vi "FPGAmain_5761.vi"() -> ()   [LabVIEW 2018]
uses:
  FPGA/DataMode.ctl
  Host/Scope/controls/host_transfer_speed.ctl
  FPGA/Input_5782/5782_Fast_PID_states.ctl
  <vilib>/Platform/TimedLoop/XDataNode/timing_clust.ctl
  <vilib>/Platform/TimedLoop/XDataNode/nitl_modes.ctl
  <vilib>/Platform/TimedLoop/XDataNode/wakeup.ctl
  <vilib>/rvi/Emulation/niFpgaGetClockAttributes.vi
  <vilib>/rvi/Emulation/niFpgaSctlEmulationGetInTimedLoop.vi
  <vilib>/rvi/Emulation/niFpgaEmulationReportErrorSimple.vi
  <vilib>/rvi/eio/common/nirviEmuTemplateMethod_errors.vi
  <vilib>/rvi/Emulation/niFpgaCriticalErrorInLSC.vi
  <vilib>/rvi/Emulation/niFpgaProcessEmulError.vi
  <vilib>/rvi/Emulation/niFpgaEmulationIsFPGAContextNoSignature.vi
  <vilib>/rvi/errors/niFpgaSetErrorForExecOnDevCompSimple.vi
  <vilib>/rvi/eio/common/nirviEmuReportErrorAndStop.vi
  <vilib>/rvi/DataTransferAndStorage/Container/Common/niFpgaContainerGetUniqueNameForEmu.vi
  <vilib>/rvi/FIFO/Fifo_Resource/nirvififoEmulationSetSize.vi
  <vilib>/rvi/FIFO/Fifo_Resource/nirviFifoEmulationQueueMgr.vi
  <instcachedir>/0/nirviFifoEmulationQueueMgr_E5CAEC123FF24DC58D834DCA3CDAA9B5.lvgen/nirviFifoEmulationQueueMgr_E5CAEC123FF24DC58D834DCA3CDAA9B5_015.vi
  <vilib>/rvi/FIFO/Fifo_Resource/nirvififoEmulationDetermineInputValidOut.vi
  <vilib>/rvi/FIFO/Fifo_Resource/nirvififoEmulationCreateLock.vi
  <vilib>/rvi/FIFO/Fifo_Resource/nirvififoEmulationObtainLock.vi
  <vilib>/rvi/FIFO/Fifo_Resource/nirvififoEmulationReleaseLock.vi
  <vilib>/rvi/occurrence/nirviWaitOnOccurrenceBase.vi
  <vilib>/rvi/errors/nirviReportUnexpectedCaseInternalError.vi
  <vilib>/rvi/errors/nirviReportUnexpectedCaseInternalError (U32).vi
  <vilib>/rvi/Memory/Memory_Emulation/niFpgaMemoryEmulationCacheClearOnFirstRun.vi
  <vilib>/rvi/Memory/Memory_Emulation/nirvimemoryEmulationManagerCache_MakeExclusive.vi
  <vilib>/rvi/Memory/Memory_Emulation/niFpgaMemoryEmulationValidateCache.vi
  <vilib>/rvi/Memory/Memory_Emulation/nirvimemoryEmulationManagerCache_InsertValue.vi
  <vilib>/Utility/error.llb/Clear Errors.vi
  <vilib>/rvi/Memory/Memory_Emulation/nirvimemoryEmulationManagerCache_ReleaseExclusive.vi
  <vilib>/rvi/Memory/Memory_Emulation/nirvimemoryEmulationManagerCache_GetValue.vi
  <vilib>/rvi/Memory/Memory_Emulation/nirvimemoryEmulationManagerCache_SetValue.vi
  <instcachedir>/0/nirviFifoEmulationQueueMgr_E5CAEC123FF24DC58D834DCA3CDAA9B5.lvgen/nirviFifoEmulationQueueMgr_E5CAEC123FF24DC58D834DCA3CDAA9B5_019.vi
  <vilib>/rvi/interface/RandomDataEmulation/niFpgaRandomDataHandleErrors.vi
  <instcachedir>/0/nirviFifoEmulationQueueMgr_E5CAEC123FF24DC58D834DCA3CDAA9B5.lvgen/nirviFifoEmulationQueueMgr_E5CAEC123FF24DC58D834DCA3CDAA9B5_025.vi
  <vilib>/rvi/interface/RandomDataEmulation/nirviRandomDataMultiElementFPGAFIFO.vi
  <instcachedir>/0/nirviRandomDataMultiElementFPGAFIFO_6740B454F3C245F78F76ED91F73FD8DB.lvgen/nirviRandomDataMultiElementFPGAFIFO_6740B454F3C245F78F76ED91F73FD8DB_000.vi
  <vilib>/eio/EIONode/EIONode.xnode
  <vilib>/Platform/TimedLoop/XDataNode/XDataNode.xnode
  <vilib>/rvi/FXPMathLib/FxpInterpret/XNode/nifxpmath_Interpret.xnode
  <vilib>/rvi/DataTransferAndStorage/Container/XNode/niFpgaContainer.xnode
  <vilib>/rvi/FIFO/Fifo_Resource/nirvififoEmulationWrite.vi
  <vilib>/rvi/DataTransferAndStorage/Register/Emulation/niFpgaRegisterEmulation.vi
  <vilib>/rvi/FIFO/Fifo_Resource/nirvififoEmulationRead.vi
  <vilib>/rvi/interface/RandomDataEmulation/nirviRandomDataFpgaReadWriteTemplate.vi
  <vilib>/rvi/interface/RandomDataEmulation/nirviRandomDataFpgaMultiElementTemplate.vi
  <vilib>/Platform/TimedLoop/XDataNode/XDNodeRunTimeDep.lvlib
panel:
  in  "Transfer speed":T1
  out "Num timeout":u32
  in  "W12 enabled":bool
  in  "Sample Clock Commit":bool
  in  "Sample Clock Select":u8
  out "SPI Idle":bool
  out "Configuration Error":bool
  out "Synthesizer Locked":bool
  out "Configured?":bool
  in  "Continuous":bool
  in  "Record length":u16=4000 caption="Samples Per Trigger" min=1 step=1
  in  "Trigger Acquisition":bool
  out "IO Module\\Trigger Input":bool
  in  "Acquisition running":bool
  in  "Simulated phase":fxp<+,64,64>[](array[numeric])=[0.0, 0.0]
  in  "Mode":T2
  in  "Phase input":fxp<+,64,64>[](array[numeric])=[0.0, 0.0, 0.0, 0.0, 0.0, 0.0, 0.0, 0.0, 0.0, 0.0, 0.0, 0.0, 0.0, 0.0, 0.0, 0.0]
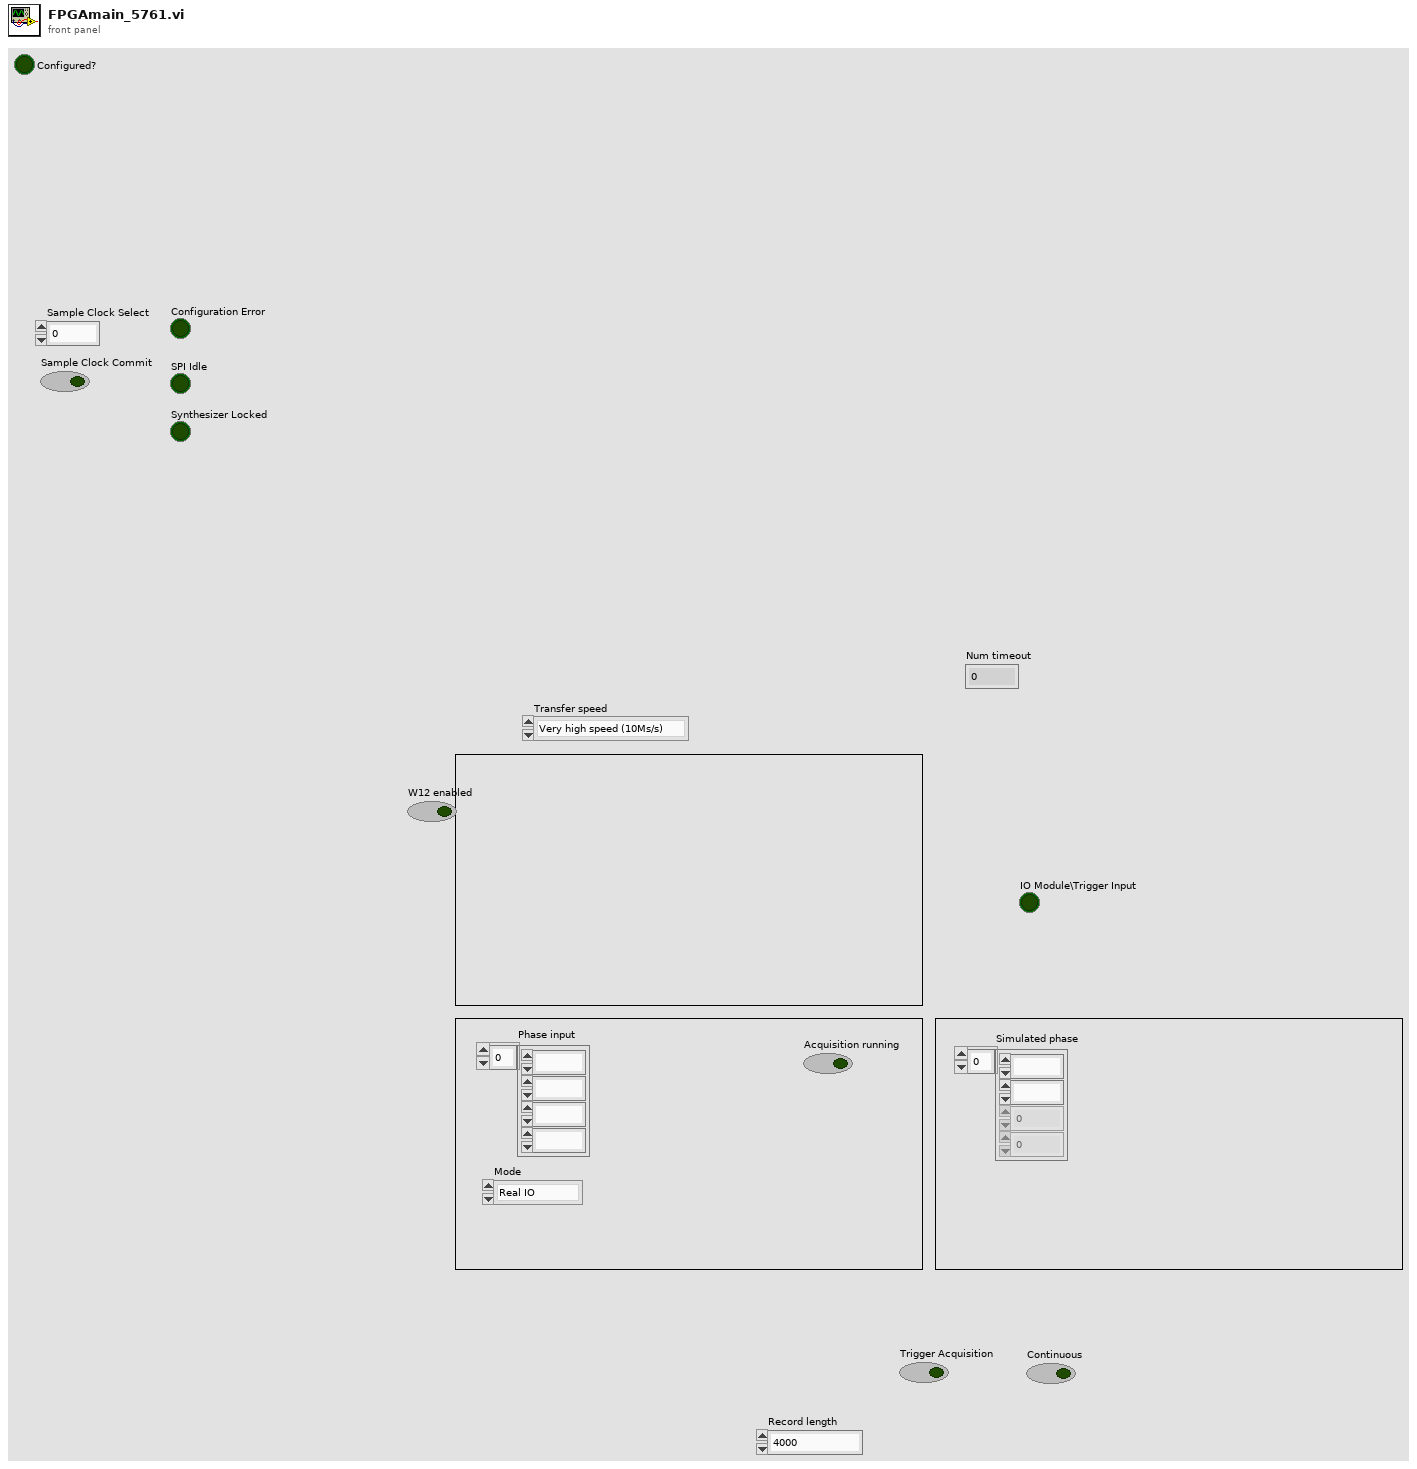
[diagram p1: front panel]
types:
  T1 = typedef "host_transfer_speed.ctl" = enum16{"Very high speed (10Ms/s)", "High speed (1Ms/s)", "Low speed (50kS/s)", "Ultra low speed (20kS/s)"}
  T2 = typedef "DataMode.ctl" = enum16{"Real IO", "Simulated"}
  T3 = typedef "5782_Fast_PID_states.ctl" = enum8{"Wait for trigger", "Acquisition", "Send record length", "Wait for output", "Quiet period"}
  T4 = typedef "XDNodeRunTimeDep.lvlib/timing_clust.ctl" = cluster{"Expected End [f-1]":u64, "Actual End [f-1]":u64, "Finished Late? [f-1]":bool, "Expected End [i-1]":u64, "Actual End [i-1]":u64, "Finished Late? [i-1]":bool, "Expected Start [i]":u64, "Actual Start [i]":u64, "Expected Start [f]":u64, "Actual Start [f]":u64, "Source Name":string, "Structure Name":string, "Period":i64, "Deadline":i64, "Offset":i64, "Start":i64, "Priority":i32, "Timeout":i32, "Mode":T5, "Wakeup Reason":T6, "Error":errorcluster, "Source Type":string, "Secondary Source Type":string, "Global End Time":u64, "Global Start Time":u64, "Frame Duration":u64, "Iteration Duration":u64, "Assigned CPU":i32, "I/O Scan Engine Mode":u32}
  T5 = typedef "XDNodeRunTimeDep.lvlib/nitl_modes.ctl" = enum32{"No Change", "Process missed periods, maintain original phase", "Discard missed periods, maintain original phase", "Process missed periods, ignore original phase", "Discard missed periods, ignore original phase"}
  T6 = typedef "XDNodeRunTimeDep.lvlib/wakeup.ctl" = enum32{"Normal", "Aborted", "Asynchronous wakeup", "Timing source error", "Timed loop error", "Timeout"}
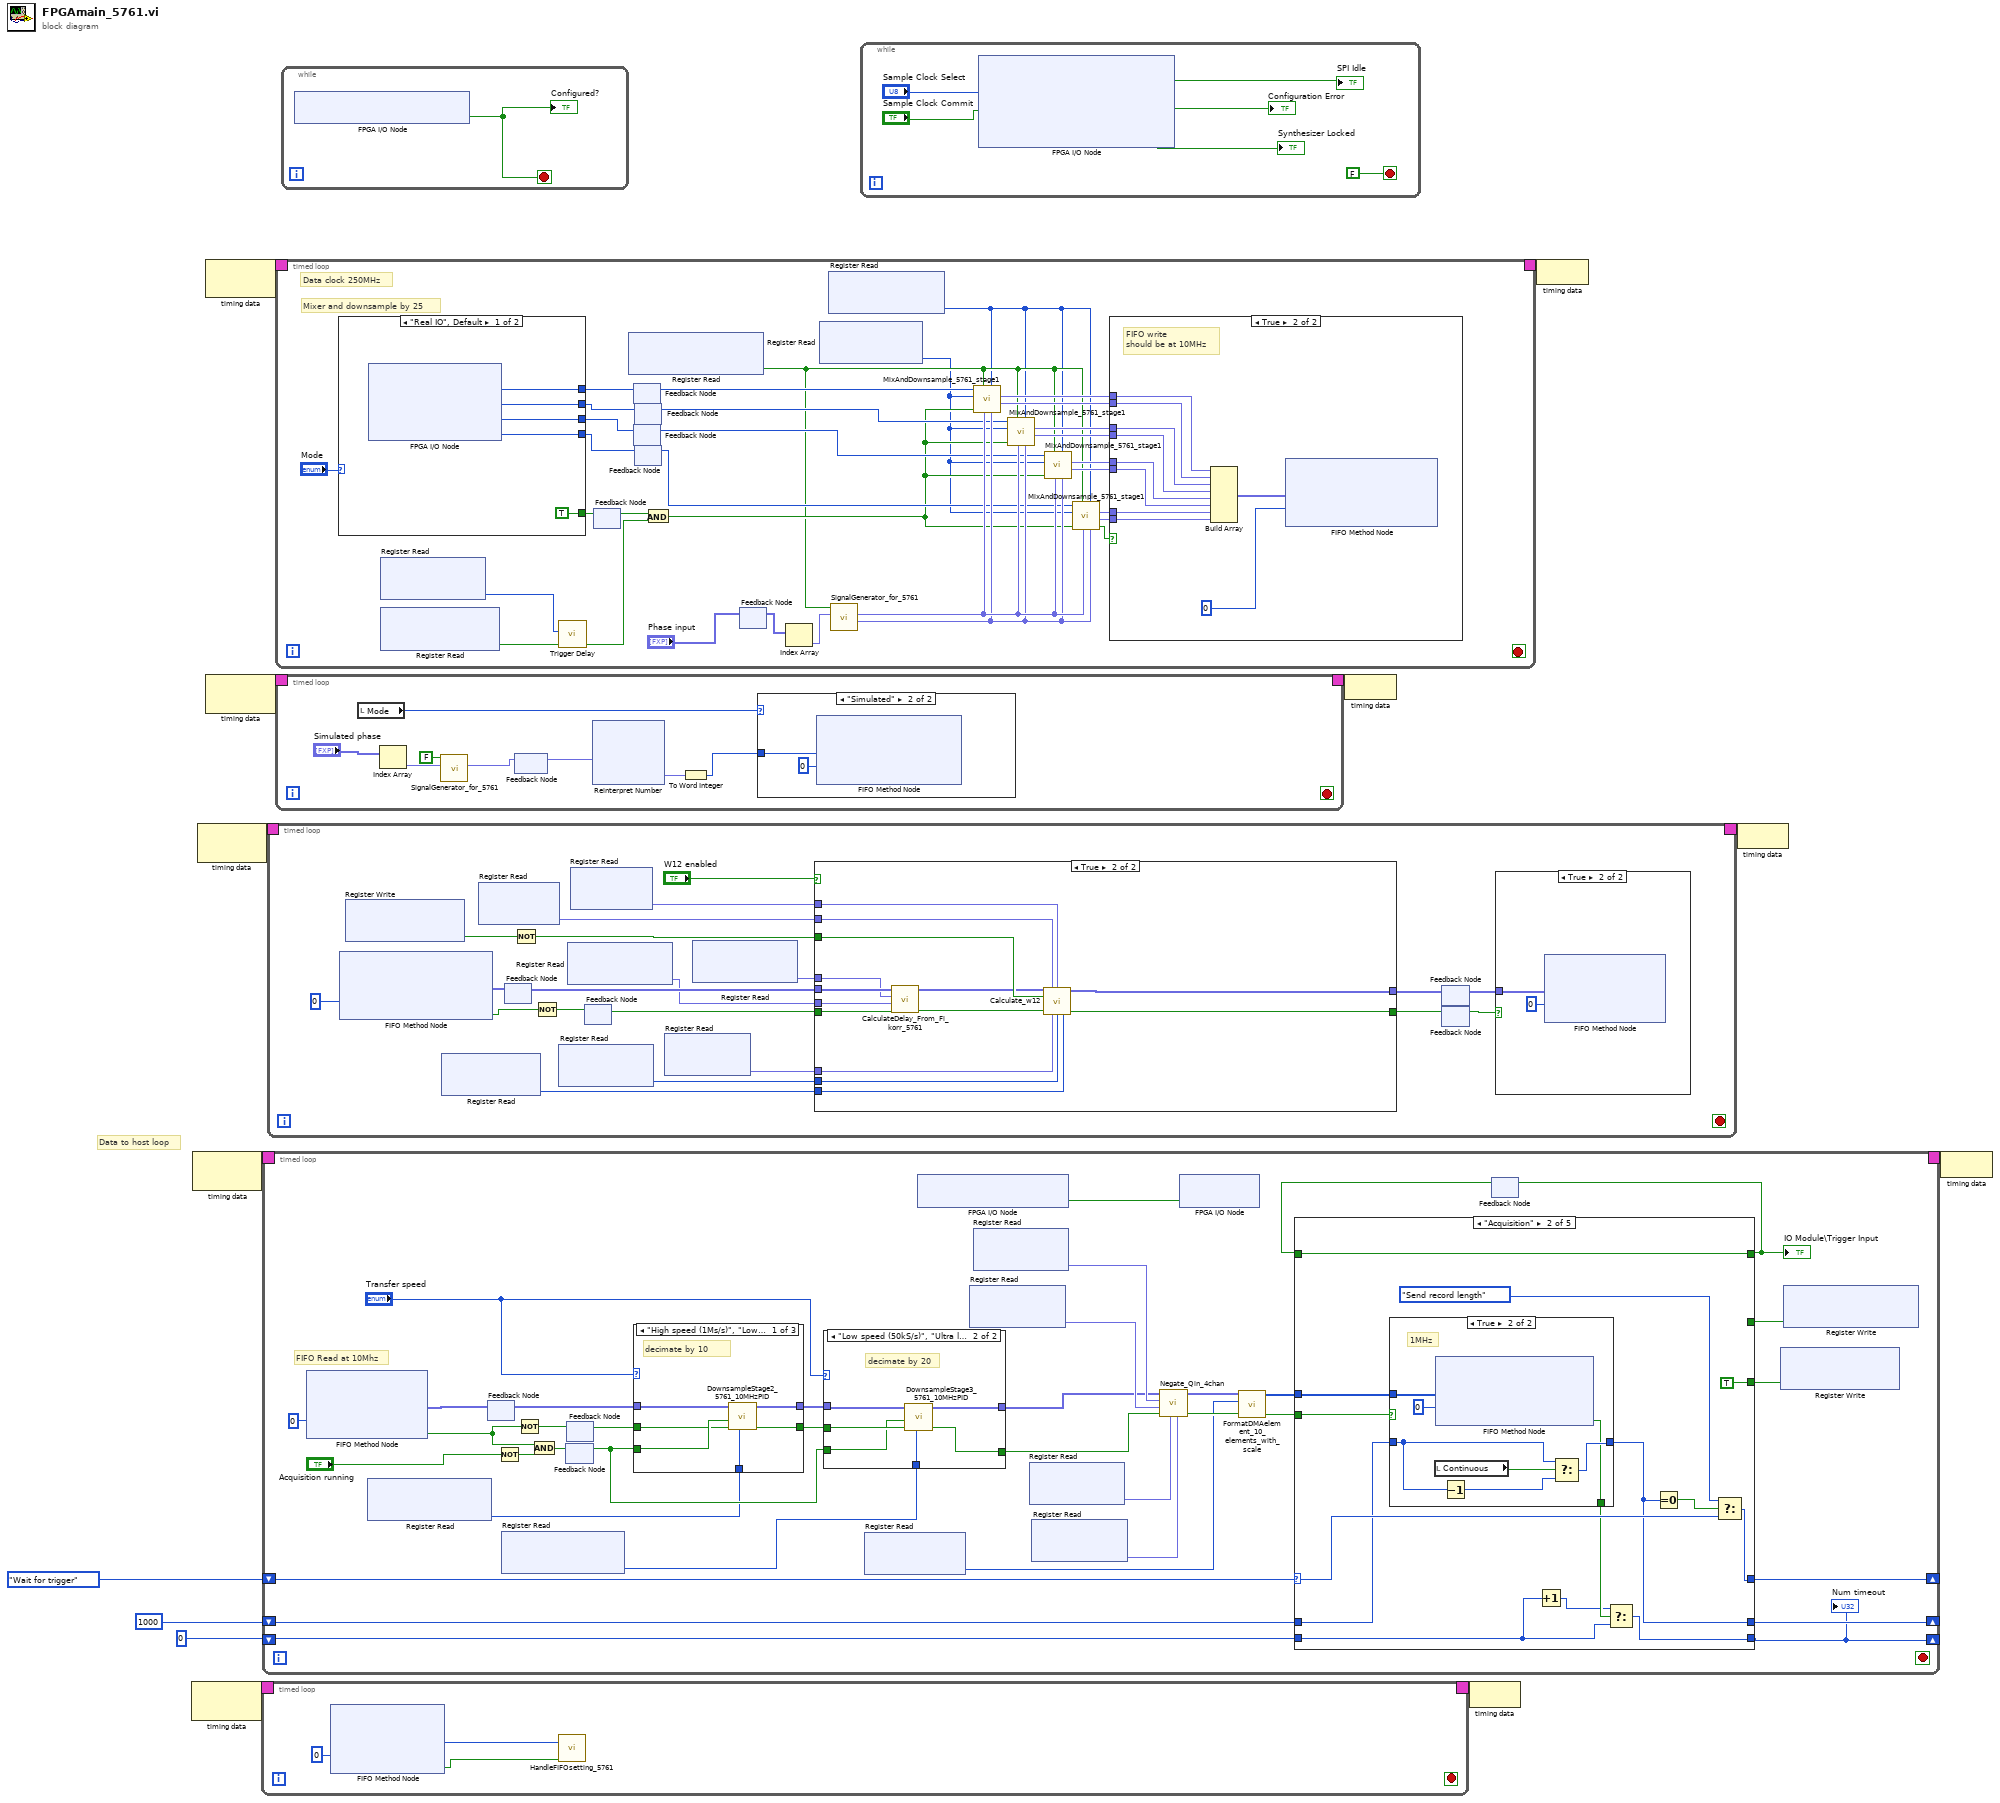
[diagram p0: block diagram]
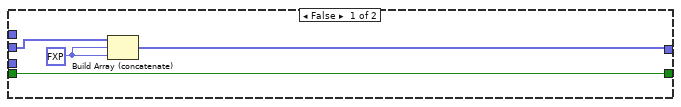
[diagram p2: hidden frame]
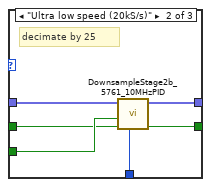
[diagram p5: hidden frame]
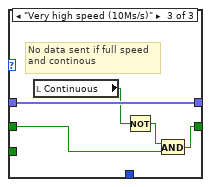
[diagram p6: hidden frame]
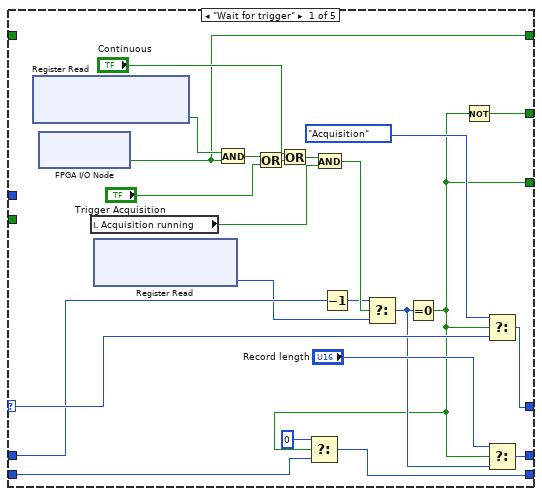
[diagram p7: hidden frame]
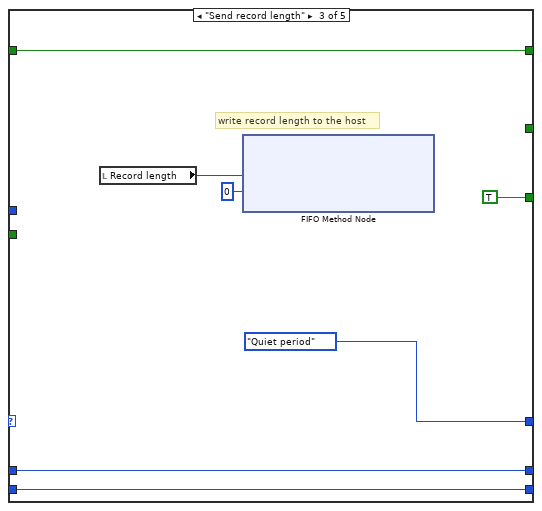
[diagram p9: hidden frame]
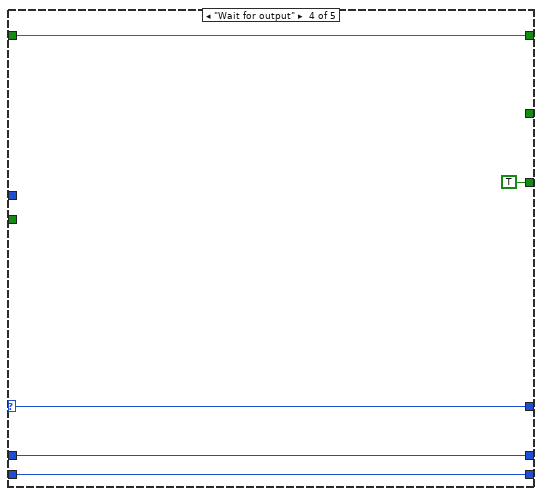
[diagram p10: hidden frame]
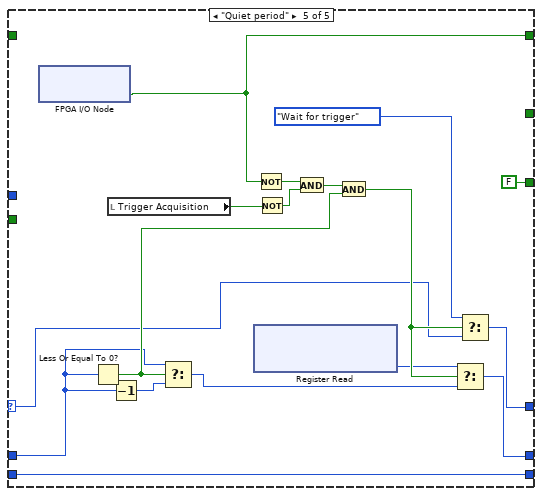
[diagram p11: hidden frame]
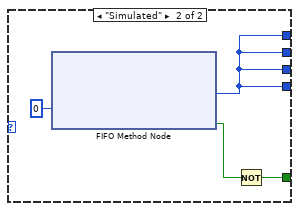
[diagram p13: hidden frame]
diagram:
  # "Data to host loop"
  n1 = node-c288() -> (w8:T4)  [unwired: 1 in]
  n2 = node-c288() -> (w6:T4)  [unwired: 1 in]
  n3 = node-c288() -> (w3:T4)  [unwired: 1 in]
  n4 = node-c288() -> (w11:T4)  [unwired: 1 in]
  n5 = node-c288() -> (w13:T4)  [unwired: 1 in]
  n6 = timed-loop {
    timing: w8 -> [_]
    timing-out: [_] -> w7
    stop <- _ stop-if-true
    n7 = xnode ("FIFO Method Node")("Timeout"=0) -> ("Element"=w15:u64, "Timed Out?"=w14:bool)  [unwired: 1 in, 1 out]
    n8 = call "HandleFIFOsetting_5761.vi"("timed out"=w14, "Value"=w15) -> ()  [unwired: 10 in]
  }
  n9 = timed-loop {
    timing: w6 -> [_]
    timing-out: [_] -> w5
    shift-right: [w53] -> _
    shift-left: 5782_Fast_PID_states."Wait for trigger" ("5782 states") -> [w55]
    shift-right: [w52] -> _
    shift-left: u16 1000 ("trigger samples") -> [w54]
    shift-right: [w20] -> _
    shift-left: u32 0 ("trigger samples") -> [w21]
    stop <- _ stop-if-true
    # "FIFO Read at 10Mhz"
    n10 = xnode ("FIFO Method Node")("Timeout"=0) -> ("Element"=w31:fxp<+/-,32,14>[], "Timed Out?"=w30:bool)  [unwired: 1 in, 1 out]
    n11 = xnode ("Register Read")() -> ("Data"=w23:u32)  [unwired: 1 in, 1 out]
    n12 = feedback #1() -> (w32:fxp<+/-,32,14>[])  [unwired: 1 in]
    n13 = feedback-in #1(w31) -> ()
    n14 = Not(x="Acquisition running") -> (.not. x?=w37:bool)
    n15 = xnode ("Register Read")() -> ("Data"=w22:u32)  [unwired: 1 in, 1 out]
    n16 = Not(x=w30) -> (.not. x?=w35:bool)
    n17 = And(x=w30, y=w37) -> (x .and. y?=w34:bool)
    n18 = feedback #2() -> (w26:bool)  [unwired: 1 in]
    n19 = feedback-in #2(w34) -> ()
    n20 = feedback #3() -> (w36:bool)  [unwired: 1 in]
    n21 = feedback-in #3(w35) -> ()
    n22 = case shown="\"High speed (1Ms/s)\", \"Low speed (50kS/s)\"" "Transfer speed" {
      tunnel: [w69 w75 w80] -> w27
      tunnel: [w68 w74 w76] -> w28
      tunnel: w32 -> [w67 w73 w80]
      tunnel: w26 -> [w66 w72 _]
      tunnel: w36 -> [w65 w71 w78]
      tunnel: w23 -> [w64 w70 _]
      frame "High speed (1Ms/s)", "Low speed (50kS/s)" {
        # "decimate by 10"
        n23 = call "DownsampleStage2_5761_10MHzPID.vi"("Count to skip"=w64, "valid in"=w65, "reset"=w66, "Data in"=w67) -> ("valid out"=w68:bool, "data out"=w69:fxp<+/-,32,14>[])  [unwired: 6 in]
      }
      frame "Ultra low speed (20kS/s)" {
        # "decimate by 25"
        n24 = call "DownsampleStage2b_5761_10MHzPID.vi"("Count to skip"=w70, "valid in"=w71, "reset"=w72, "Data in"=w73) -> ("valid out"=w74:bool, "data out"=w75:fxp<+/-,32,14>[])  [unwired: 6 in]
      }
      frame "Very high speed (10Ms/s)" {
        # "No data sent if full speed\nand continous"
        n25 = local read "Continuous"() -> (w79:bool)
        n26 = Not(x=w79) -> (.not. x?=w77:bool)
        n27 = And(x=w77, y=w78) -> (x .and. y?=w76:bool)
      }
    }
    n28 = case shown="\"Low speed (50kS/s)\", \"Ultra low speed (20kS/s)\"" "Transfer speed" {
      tunnel: [w56 w63] -> w25
      tunnel: [w57 w62] -> w24
      tunnel: w26 -> [_ w60]
      tunnel: w28 -> [w57 w61]
      tunnel: w27 -> [w56 w59]
      tunnel: w22 -> [_ w58]
      frame "Very high speed (10Ms/s)", Default {
      }
      frame "Low speed (50kS/s)", "Ultra low speed (20kS/s)" {
        # "decimate by 20"
        n29 = call "DownsampleStage3_5761_10MHzPID.vi"("Count to skip"=w58, "valid in"=w61, "reset"=w60, "Data in"=w59) -> ("valid out"=w62:bool, "data out"=w63:fxp<+/-,32,14>[])  [unwired: 6 in]
      }
    }
    n30 = xnode ("Register Read")() -> ("Data"=w38:u16)  [unwired: 1 in, 1 out]
    n31 = xnode "FPGA I/O Node"() -> ("IO Module\\Trigger Input"=w39:bool)  [unwired: 1 in, 1 out]
    n32 = xnode ("Register Read")() -> ("Data"=w44:fxp<+/-,32,14>)  [unwired: 1 in, 1 out]
    n33 = xnode ("Register Read")() -> ("Data"=w45:fxp<+/-,32,14>)  [unwired: 1 in, 1 out]
    n34 = xnode ("Register Read")() -> ("Data"=w43:fxp<+/-,32,14>)  [unwired: 1 in, 1 out]
    n35 = xnode ("Register Read")() -> ("Data"=w42:fxp<+/-,32,14>)  [unwired: 1 in, 1 out]
    n36 = call "Negate_Qin_4chan.vi"("DC offset chan 3"=w42, "DC offset chan 2"=w43, "valid in"=w24, "DC offset chan 1"=w44, "DC offset chan 0"=w45, "Data in"=w25) -> ("valid out"=w46:bool, "Data out"=w47:fxp<+/-,32,14>[])  [unwired: 4 in]
    n37 = xnode "FPGA I/O Node"("PXI_Trig0"=w39) -> ()  [unwired: 1 in, 1 out]
    n38 = call "FormatDMAelement_10_elements_with_scale.vi"("valid in"=w46, "factor"=w38, "Data in"=w47) -> ("valid out"=w50:bool, "Values"=w49:u64[])  [unwired: 7 in]
    n39 = feedback #4() -> (w40:bool)  [unwired: 1 in]
    n40 = case shown="\"Acquisition\"" w55 {
      selector: w55 -> [w103 w117 _ w135 w141]
      tunnel: w54 -> [w94 w114 w127 w134 w142]
      tunnel: [w102 w116 5782_Fast_PID_states."Quiet period" ("5782 states") w135 w153] -> w53
      tunnel: [w101 w111 w127 w134 w154] -> w52
      tunnel: w49 -> [_ w112 _ _ _]
      tunnel: w50 -> [_ w113 _ _ _]
      tunnel: [w83 TRUE TRUE ("5782 triggered") TRUE ("5782 triggered") FALSE ("5782 triggered")] -> w51
      tunnel: [w85 w110 w129 w136 w139] -> w41
      tunnel: w40 -> [_ w110 w129 w136 _]
      tunnel: [w89 _ _ _ _] -> w48
      tunnel: w21 -> [w84 w105 w126 w133 w138]
      tunnel: [w81 w104 w126 w133 w138] -> w20
      frame "Wait for trigger" {
        n41 = xnode ("Register Read")() -> ("Data"=w87:bool)  [unwired: 1 in, 1 out]
        n42 = xnode "FPGA I/O Node"() -> ("PXI_Trig0"=w85:bool)  [unwired: 1 in, 1 out]
        n43 = local read "Acquisition running"() -> (w97:bool)
        n44 = xnode ("Register Read")() -> ("Data"=w90:u16)  [unwired: 1 in, 1 out]
        n45 = And(x=w87, y=w85) -> (x .and. y?=w86:bool)
        n46 = Or(x=w86, y="Trigger Acquisition") -> (x .or. y?=w93:bool)
        n47 = Or(x="Continuous", y=w93) -> (x .or. y?=w91:bool)
        n48 = And(x=w91, y=w97) -> (x .and. y?=w98:bool)
        n49 = Decrement(x=w94) -> (x-1=w95:u16)
        n50 = Select(t=w95, s=w98, f=w90) -> (s? t:f=w96:u16)
        n51 = Equal To 0?(x=w96) -> (x = 0?=w83:bool)
        n52 = Select(t=u32 0, s=w83, f=w84) -> (s? t:f=w81:u32)
        n53 = Not(x=w83) -> (.not. x?=w89:bool)
        n54 = Select(t=5782_Fast_PID_states."Acquisition" ("5782 states"), s=w83, f=w103) -> (s? t:f=w102:T3)
        n55 = Select(t="Record length", s=w83, f=w96) -> (s? t:f=w101:u16)
      }
      frame "Acquisition" {
        n56 = case shown="True" w113 {
          tunnel: w112 -> [_ w125]
          tunnel: [w118 w122] -> w111
          tunnel: w114 -> [w118 w120]
          tunnel: [_ w119] -> w107
          frame False {
          }
          frame True {
            # "1MHz"
            n57 = local read "Continuous"() -> (w123:bool)
            n58 = xnode ("FIFO Method Node")("Element"=w125, "Timeout"=0) -> ("Timed Out?"=w119:bool)  [unwired: 1 in, 1 out]
            n59 = Decrement(x=w120) -> (x-1=w121:u16)
            n60 = Select(t=w120, s=w123, f=w121) -> (s? t:f=w122:u16)
          }
        }
        n61 = Increment(x=w105) -> (x+1=w106:u32)
        n62 = Select(t=w106, s=w107, f=w105) -> (s? t:f=w104:u32)
        n63 = Equal To 0?(x=w111) -> (x = 0?=w115:bool)
        n64 = Select(t=5782_Fast_PID_states."Send record length" ("5782 states"), s=w115, f=w117) -> (s? t:f=w116:T3)
      }
      frame "Send record length" {
        # "write record length to the host"
        n65 = local read "Record length"() -> (w131:u16)
        n66 = xnode ("FIFO Method Node")("Element"=w131, "Timeout"=0) -> ()  [unwired: 1 in, 2 out]
      }
      frame "Wait for output" {
      }
      frame "Quiet period" {
        n67 = xnode "FPGA I/O Node"() -> ("PXI_Trig0"=w139:bool)  [unwired: 1 in, 1 out]
        n68 = Less Or Equal To 0?(x=w142) -> (x <= 0?=w145:bool)
        n69 = local read "Trigger Acquisition"() -> (w151:bool)
        n70 = Decrement(x=w142) -> (x-1=w146:u16)
        n71 = Select(t=w142, s=w145, f=w146) -> (s? t:f=w144:u16)
        n72 = xnode ("Register Read")() -> ("Data"=w143:u16)  [unwired: 1 in, 1 out]
        n73 = Not(x=w139) -> (.not. x?=w150:bool)
        n74 = Not(x=w151) -> (.not. x?=w149:bool)
        n75 = And(x=w150, y=w149) -> (x .and. y?=w148:bool)
        n76 = And(x=w148, y=w145) -> (x .and. y?=w152:bool)
        n77 = Select(t=w143, s=w152, f=w144) -> (s? t:f=w154:u16)
        n78 = Select(t=5782_Fast_PID_states."Wait for trigger" ("5782 states"), s=w152, f=w141) -> (s? t:f=w153:T3)
      }
    }
    "IO Module\\Trigger Input" <- w41
    "Num timeout" <- w20
    n79 = feedback-in #4(w41) -> ()
    n80 = xnode ("Register Write")("Data"=w51) -> ()  [unwired: 1 in, 1 out]
    n81 = xnode ("Register Write")("Data"=w48) -> ()  [unwired: 1 in, 1 out]
  }
  n82 = timed-loop {
    timing: w3 -> [_]
    timing-out: [_] -> w2
    stop <- _ stop-if-true
    n83 = xnode ("FIFO Method Node")("Timeout"=0) -> ("Element"=w174:fxp<+/-,32,14>[], "Timed Out?"=w173:bool)  [unwired: 1 in, 1 out]
    n84 = xnode ("Register Write")() -> ("Data"=w170:bool)  [unwired: 1 in, 1 out]
    n85 = xnode ("Register Read")() -> ("Data"=w160:i32)  [unwired: 1 in, 1 out]
    n86 = xnode ("Register Read")() -> ("Data"=w164:fxp<+/-,32,12>)  [unwired: 1 in, 1 out]
    n87 = feedback #5() -> (w172:fxp<+/-,32,14>[])  [unwired: 1 in]
    n88 = feedback-in #5(w174) -> ()
    n89 = Not(x=w170) -> (.not. x?=w169:bool)
    n90 = Not(x=w173) -> (.not. x?=w175:bool)
    n91 = xnode ("Register Read")() -> ("Data"=w159:i32)  [unwired: 1 in, 1 out]
    n92 = xnode ("Register Read")() -> ("Data"=w157:fxp<+/-,32,4>)  [unwired: 1 in, 1 out]
    n93 = xnode ("Register Read")() -> ("Data"=w163:fxp<+/-,32,14>)  [unwired: 1 in, 1 out]
    n94 = feedback #6() -> (w171:bool)  [unwired: 1 in]
    n95 = feedback-in #6(w175) -> ()
    n96 = xnode ("Register Read")() -> ("Data"=w161:fxp<+/-,32,26>)  [unwired: 1 in, 1 out]
    n97 = xnode ("Register Read")() -> ("Data"=w158:fxp<+/-,32,4>)  [unwired: 1 in, 1 out]
    n98 = case shown="True" "W12 enabled" {
      tunnel: w172 -> [w179 w186]
      tunnel: w171 -> [w180 w184]
      tunnel: w169 -> [_ w194]
      tunnel: [w177 w193] -> w168
      tunnel: [w180 w192] -> w167
      tunnel: w164 -> [_ w191]
      tunnel: w163 -> [_ w190]
      tunnel: w161 -> [_ w189]
      tunnel: w160 -> [_ w188]
      tunnel: w159 -> [_ w187]
      tunnel: w158 -> [_ w182]
      tunnel: w157 -> [_ w181]
      frame False {
        w178 = fxp<+/-,32,14> 0.0 ("Q out")
        n99 = Build Array (concatenate)(w179, w178, w178) -> (w177:fxp<+/-,32,14>[])
      }
      frame True {
        n100 = call "CalculateDelay_From_Fi_korr_5761.vi"("input valid"=w184, "fi_korr ch3"=w181, "fi_korr ch1"=w182, "Data in"=w186) -> ("output valid"=w183:bool, "Data out"=w185:fxp<+/-,32,14>[])  [unwired: 6 in]
        n101 = call "Calculate_w12.vi"("Data in"=w185, "w12_a"=w191, "w12_b"=w190, "reset"=w194, "valid in"=w183, "1/dt"=w189, "dw scale"=w187, "w12 scale"=w188) -> ("data out"=w193:fxp<+/-,32,14>[], "valid out"=w192:bool)  [unwired: 4 in, 2 out]
      }
    }
    n102 = feedback #7() -> (w165:fxp<+/-,32,14>[])  [unwired: 1 in]
    n103 = feedback-in #7(w168) -> ()
    n104 = feedback #8() -> (w166:bool)  [unwired: 1 in]
    n105 = feedback-in #8(w167) -> ()
    n106 = case shown="True" w166 {
      tunnel: w165 -> [_ w196]
      frame False {
      }
      frame True {
        n107 = xnode ("FIFO Method Node")("Element"=w196, "Timeout"=0) -> ()  [unwired: 1 in, 2 out]
      }
    }
  }
  n108 = timed-loop {
    timing: w11 -> [_]
    timing-out: [_] -> w10
    stop <- _ stop-if-true
    # "Mixer and downsample by 25"
    # "Data clock 250MHz"
    n109 = case shown="\"Real IO\", Default" "Mode" {
      tunnel: [TRUE w247] -> w229
      tunnel: [w244 w246] -> w226
      tunnel: [w243 w246] -> w225
      tunnel: [w242 w246] -> w224
      tunnel: [w241 w246] -> w223
      frame "Real IO", Default {
        n110 = xnode "FPGA I/O Node"() -> ("IO Module\\AI 0 Data"=w244:i16, "IO Module\\AI 1 Data"=w243:i16, "IO Module\\AI 2 Data"=w242:i16, "IO Module\\AI 3 Data"=w241:i16)  [unwired: 4 in, 4 out]
      }
      frame "Simulated" {
        n111 = xnode ("FIFO Method Node")("Timeout"=0) -> ("Element"=w246:i16, "Timed Out?"=w248:bool)  [unwired: 1 in, 1 out]
        n112 = Not(x=w248) -> (.not. x?=w247:bool)
      }
    }
    n113 = xnode ("Register Read")() -> ("Data"=w214:u32)  [unwired: 1 in, 1 out]
    n114 = xnode ("Register Read")() -> ("Data"=w213:bool)  [unwired: 1 in, 1 out]
    n115 = call "Trigger Delay.vi"("input valid"=w213, "Count to skip"=w214) -> ("output valid"=w212:bool)  [unwired: 9 in]
    n116 = feedback #9() -> (w228:bool)  [unwired: 1 in]
    n117 = feedback-in #9(w229) -> ()
    n118 = xnode ("Register Read")() -> ("Data"=w201:bool)  [unwired: 1 in, 1 out]
    n119 = feedback #10() -> (w222:i16)  [unwired: 1 in]
    n120 = feedback-in #10(w226) -> ()
    n121 = feedback #11() -> (w216:i16)  [unwired: 1 in]
    n122 = feedback-in #11(w224) -> ()
    n123 = feedback #12() -> (w217:i16)  [unwired: 1 in]
    n124 = feedback-in #12(w225) -> ()
    n125 = feedback #13() -> (w215:i16)  [unwired: 1 in]
    n126 = feedback-in #13(w223) -> ()
    n127 = And(x=w228, y=w212) -> (x .and. y?=w202:bool)
    n128 = feedback #14() -> (w221:fxp<+,64,64>[])  [unwired: 1 in]
    n129 = feedback-in #14("Phase input") -> ()
    n130 = Index Array(array=w221) -> (element=w220:fxp<+,64,64>)  [unwired: 1 in]
    n131 = xnode ("Register Read")() -> ("Data"=w200:u16)  [unwired: 1 in, 1 out]
    n132 = xnode ("Register Read")() -> ("Data"=w199:u32)  [unwired: 1 in, 1 out]
    n133 = call "SignalGenerator_for_5761.vi"("phase"=w220, "Reset"=w201) -> ("Cos"=w218:fxp<+/-,16,0>, "Sin"=w219:fxp<+/-,16,0>)  [unwired: 7 in, 1 out]
    n134 = call "MixAndDownsample_5761_stage1.vi"("cosine"=w218, "Count to skip"=w199, "sine"=w219, "reset"=w201, "Input Valid (T)"=w202, "factor"=w200, "Analog in"=w222) -> ("Q out"=w209:fxp<+/-,32,14>, "I out"=w210:fxp<+/-,32,14>)  [unwired: 2 in, 1 out]
    n135 = call "MixAndDownsample_5761_stage1.vi"("cosine"=w218, "Count to skip"=w199, "sine"=w219, "reset"=w201, "Input Valid (T)"=w202, "factor"=w200, "Analog in"=w217) -> ("Q out"=w207:fxp<+/-,32,14>, "I out"=w208:fxp<+/-,32,14>)  [unwired: 2 in, 1 out]
    n136 = call "MixAndDownsample_5761_stage1.vi"("cosine"=w218, "Count to skip"=w199, "sine"=w219, "reset"=w201, "Input Valid (T)"=w202, "factor"=w200, "Analog in"=w216) -> ("Q out"=w205:fxp<+/-,32,14>, "I out"=w206:fxp<+/-,32,14>)  [unwired: 2 in, 1 out]
    n137 = call "MixAndDownsample_5761_stage1.vi"("cosine"=w218, "Count to skip"=w199, "sine"=w219, "reset"=w201, "Input Valid (T)"=w202, "factor"=w200, "Analog in"=w215) -> ("data valid"=w211:bool, "Q out"=w203:fxp<+/-,32,14>, "I out"=w204:fxp<+/-,32,14>)  [unwired: 2 in]
    n138 = case shown="True" w211 {
      tunnel: w210 -> [_ w238]
      tunnel: w209 -> [_ w237]
      tunnel: w208 -> [_ w236]
      tunnel: w207 -> [_ w235]
      tunnel: w206 -> [_ w234]
      tunnel: w205 -> [_ w233]
      tunnel: w204 -> [_ w232]
      tunnel: w203 -> [_ w231]
      frame False {
      }
      frame True {
        # "FIFO write\nshould be at 10MHz"
        n139 = Build Array(w238, w237, w236, w235, w234, w233, w232, w231) -> (w240:fxp<+/-,32,14>[])
        n140 = xnode ("FIFO Method Node")("Element"=w240, "Timeout"=0) -> ()  [unwired: 1 in, 2 out]
      }
    }
  }
  n141 = timed-loop {
    timing: w13 -> [_]
    timing-out: [_] -> w12
    stop <- _ stop-if-true
    n142 = local read "Mode"() -> (w259:T2)
    n143 = Index Array(array="Simulated phase") -> (element=w258:fxp<+,64,64>)  [unwired: 1 in]
    n144 = call "SignalGenerator_for_5761.vi"("phase"=w258, "Reset"=FALSE) -> ("Sin"=w253:fxp<+/-,16,0>)  [unwired: 7 in, 2 out]
    n145 = feedback #15() -> (w254:fxp<+/-,16,0>)  [unwired: 1 in]
    n146 = feedback-in #15(w253) -> ()
    n147 = xnode "Reinterpret Number"("x"=w254) -> ("y"=w255:fxp<+/-,16,13>)
    n148 = To Word Integer(number=w255) -> (16bit integer=w252:i16)
    n149 = case shown="\"Simulated\"" w259 {
      tunnel: w252 -> [_ w260]
      frame "Real IO", Default {
      }
      frame "Simulated" {
        n150 = xnode ("FIFO Method Node")("Element"=w260, "Timeout"=0) -> ()  [unwired: 1 in, 2 out]
      }
    }
  }
  n151 = while {
    stop <- w264 stop-if-true
    n152 = xnode "FPGA I/O Node"() -> ("IO Module\\Initialization Done"=w264:bool)  [unwired: 1 in, 1 out]
    "Configured?" <- w264
  }
  n153 = while {
    stop <- FALSE stop-if-true
    n154 = xnode "FPGA I/O Node"("IO Module\\Sample Clock Select"="Sample Clock Select", "IO Module\\Sample Clock Commit"="Sample Clock Commit") -> ("IO Module\\SPI Idle"=→"SPI Idle":bool, "IO Module\\Configuration Error"=→"Configuration Error":bool, "IO Module\\Synthesizer Locked"=→"Synthesizer Locked":bool)  [unwired: 5 in, 5 out]
  }
  n155 = node-c288(w12) -> ()
  n156 = node-c288(w7) -> ()
  n157 = node-c288(w10) -> ()
  n158 = node-c288(w2) -> ()
  n159 = node-c288(w5) -> ()
